vi "0.vi"(10 "数值":u8) -> ()   [LabVIEW 2018]
uses:
  <vilib>/rvi/eio/common/nirviEmuTemplateMethod_errors.vi
  <vilib>/eio/EIONode/EIONode.xnode
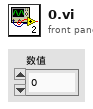
[diagram p1: front panel]
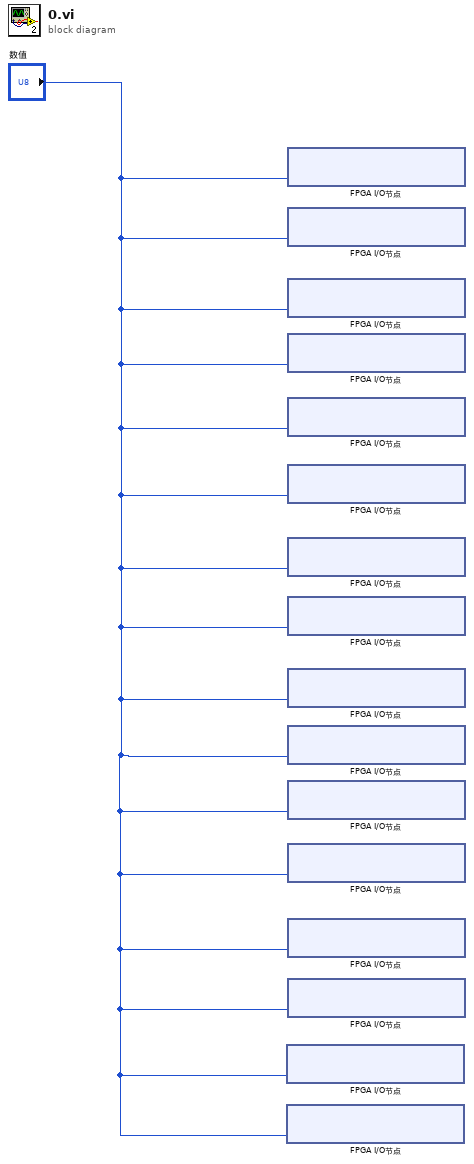
[diagram p0: block diagram]
diagram:
  n1 = xnode "FPGA I/O节点"("Connector3/DIOPORT2"="数值") -> ()  [unwired: 1 in, 1 out]
  n2 = xnode "FPGA I/O节点"("Connector3/DIOPORT4"="数值") -> ()  [unwired: 1 in, 1 out]
  n3 = xnode "FPGA I/O节点"("Connector0/DIOPORT0"="数值") -> ()  [unwired: 1 in, 1 out]
  n4 = xnode "FPGA I/O节点"("Connector0/DIOPORT1"="数值") -> ()  [unwired: 1 in, 1 out]
  n5 = xnode "FPGA I/O节点"("Connector0/DIOPORT2"="数值") -> ()  [unwired: 1 in, 1 out]
  n6 = xnode "FPGA I/O节点"("Connector0/DIOPORT3"="数值") -> ()  [unwired: 1 in, 1 out]
  n7 = xnode "FPGA I/O节点"("Connector1/DIOPORT0"="数值") -> ()  [unwired: 1 in, 1 out]
  n8 = xnode "FPGA I/O节点"("Connector1/DIOPORT1"="数值") -> ()  [unwired: 1 in, 1 out]
  n9 = xnode "FPGA I/O节点"("Connector1/DIOPORT2"="数值") -> ()  [unwired: 1 in, 1 out]
  n10 = xnode "FPGA I/O节点"("Connector2/DIOPORT3"="数值") -> ()  [unwired: 1 in, 1 out]
  n11 = xnode "FPGA I/O节点"("Connector2/DIOPORT0"="数值") -> ()  [unwired: 1 in, 1 out]
  n12 = xnode "FPGA I/O节点"("Connector2/DIOPORT1"="数值") -> ()  [unwired: 1 in, 1 out]
  n13 = xnode "FPGA I/O节点"("Connector2/DIOPORT2"="数值") -> ()  [unwired: 1 in, 1 out]
  n14 = xnode "FPGA I/O节点"("Connector2/DIOPORT3"="数值") -> ()  [unwired: 1 in, 1 out]
  n15 = xnode "FPGA I/O节点"("Connector3/DIOPORT0"="数值") -> ()  [unwired: 1 in, 1 out]
  n16 = xnode "FPGA I/O节点"("Connector3/DIOPORT1"="数值") -> ()  [unwired: 1 in, 1 out]
